vi "_Yt07_Waiting.vi"(11 "YTESTER测试数据":T1 caption="不要修改！") -> (3 "YTESTER结论":T2)   [LabVIEW 2017]
doc: "VIDescription=等待一段时间，可用StopFlag终止等待（每100ms检测停止信号）。\nVIClassID=YT_SSTEPFLAG_WAIT"
uses:
  YtCommon.lvlibp/yt`Step StepBaseInput.ctl
  YtCommon.lvlibp/yt`Step StepResult.ctl
  YtCommon.lvlibp/yt`Step TestData.ctl
  YtCommon.lvlibp/yt`Step System Queue.ctl
  YtCommon.lvlibp
panel:
  in  "YTESTER开放参数":cluster{"YTESTER_BaseInput":T3, "等待（秒）":dbl}={"YTESTER_BaseInput"={"isTest"=FALSE, "isSkip"=FALSE, "StepName"="等待", "OnPass"=enum."Next", "OnFail"=enum."Next", "ReTestNumber"=0.0}, "等待（秒）"=1.0}
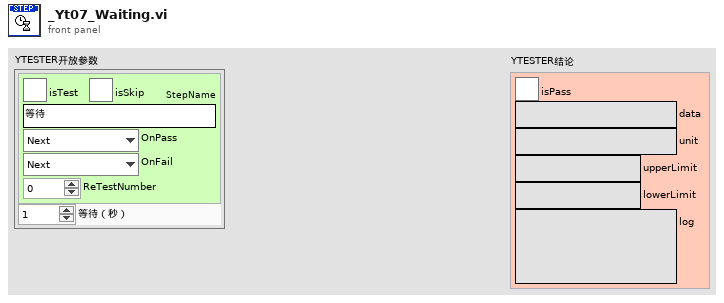
[diagram p1: front panel]
types:
  T1 = typedef "YtCommon.lvlibp/yt`Step TestData.ctl" = cluster{"Socket(From1)":i32, "SN":refnum<notifier>, "StopFlagRef":refnum<notifier>, "YT System Queue":refnum<queue>}
  T2 = typedef "YtCommon.lvlibp/yt`Step StepResult.ctl" = cluster{"isPass":bool, "data":string, "unit":string, "upperLimit":string, "lowerLimit":string, "log":string}
  T3 = typedef "YtCommon.lvlibp/yt`Step StepBaseInput.ctl" = cluster{"isTest":bool, "isSkip":bool, "StepName":string, "OnPass":enum16{"Next", "ToOVER", "Terminate"}, "OnFail":enum16{"Next", "ToOVER", "Terminate"}, "ReTestNumber":dbl}
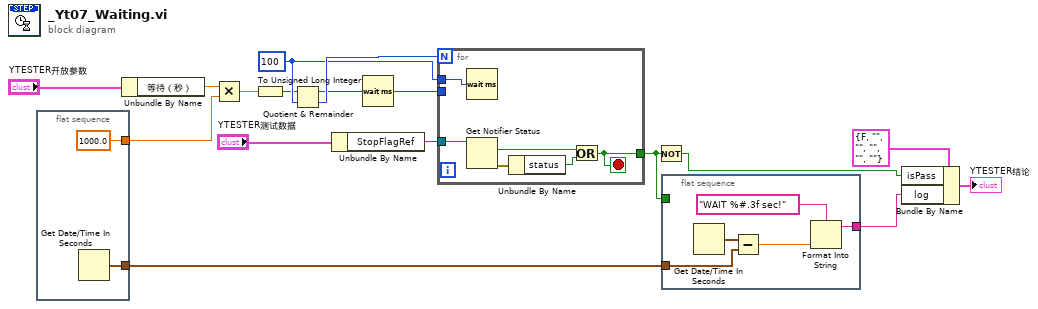
[diagram p0: block diagram]
diagram:
  w13 = u32 100 ("y")
  n1 = flat-sequence {
    tunnel: [1000.0 ("y")] -> w4
    tunnel: [w18] -> w2
    frame #0 {
      n2 = Get Date/Time In Seconds() -> (seconds since 1Jan1904=w18:timestamp)
    }
  }
  n3 = Unbundle By Name("YTESTER开放参数") -> ("等待（秒）"=w16:dbl)
  n4 = Multiply(x=w16, y=w4) -> (x*y=w15:dbl)
  n5 = To Unsigned Long Integer(number=w15) -> (unsigned 32bit integer=w12:u32)
  n6 = Quotient & Remainder(x=w12, y=w13) -> (x-y*floor(x/y)=w6:u32, floor(x/y)=w14:u32)
  n7 = Unbundle By Name("YTESTER测试数据") -> ("StopFlagRef"=w11:refnum<notifier>)
  n8 = Wait (ms)(milliseconds to wait=w6) -> (millisecond timer value=w5:u32)
  n9 = for {
    N: w14 -> [_]
    tunnel: w13 -> [w25]
    tunnel: w5 -> [_]
    tunnel: w11 -> [w24]
    tunnel: [w20] -> w1
    stop <- w20 stop-if-true
    n10 = Wait (ms)(milliseconds to wait=w25) -> ()  [unwired: 1 out]
    n11 = Get Notifier Status(notifier=w24) -> (current notification=w23:bool, error out=w22:errorcluster)  [unwired: 1 in, 3 out]
    n12 = Unbundle By Name(w22) -> ("status"=w21:bool)
    n13 = Or(x=w23, y=w21) -> (x .or. y?=w20:bool)
  }
  n14 = Not(x=w1) -> (.not. x?=w7:bool)
  n15 = flat-sequence {
    tunnel: [w26] -> w3
    tunnel: w2 -> [w29]
    tunnel: w1 -> [_]
    frame #0 {
      n16 = Get Date/Time In Seconds() -> (seconds since 1Jan1904=w30:timestamp)
      n17 = Subtract(x=w30, y=w29) -> (x-y=w28:dbl)
      n18 = Format Into String(format string="WAIT %#.3f sec!", w28) -> (resulting string=w26:string)  [unwired: 2 in, 1 out]
    }
  }
  n19 = Bundle By Name(cluster=T2 {"isPass"=FALSE, "data"="", "unit"="", "upperLimit"="", "lowerLimit"="", "log"=""} ("Result"), "isPass"=w7, "log"=w3) -> (→"YTESTER结论":T2)
